vi "grabber_framescan.vi"() -> ()   [LabVIEW 2010]
uses:
  command_enum.ctl
  status_enum.ctl
  FPGAWrapperMH120124FrameScan_PXI7813R/settings_cluster_framescan.ctl
  common_typedefs/channels_cluster.ctl
  fpgaVIsAndControls/DDS_board_init_cluster.ctl
  fpgaVIsAndControls/gate_cluster.ctl
  common_typedefs/gate_parameters_cluster.ctl
  <vilib>/rvi/interface/nirviReadWriteControl/nirviReadWriteControl.xnode
  <vilib>/rvi/interface/common/niFpgaNodeNameForErrorReporting.ctl
  <vilib>/rvi/errors/niLvFpgaWhatHappensToTopLevelVI.ctl
  <vilib>/dex/Flush And Wait Empty Condition.ctl
  <vilib>/rvi/interface/nirviMethod/nirviMethod.xnode
  <vilib>/rvi/interface/nirviCloseFPGA/nirviCloseFPGA.xnode
  <vilib>/Utility/error.llb/Error Cluster From Error Code.vi
  <vilib>/rvi/errors/niLvFpgaAdjustHostInterfaceError.vi
  <vilib>/FPGAPlugInAG/Dynamic/niLvFpga_Close_Dynamic.vi
  NiFpgaLv.dll
panel:
  out "stop":bool
  out "read size":u32
  out "Elements Remaining 1":u32
  out "element":T1 {"DDS board initialization parameters"."Modus" scale=0.0..4.0}
  out "current status":T6
  out "pixel no.":i64
  out "last command_not_acq":T7
  out "FIFO overflow?":bool
  out "last command?":T7
  out "error out":errorcluster
  # "FSK"
  # "Ramped"
  # "FSK"
  # "Chirp Modus"
  # "Unramped"
  # "BPSK"
  # "Single Tone"
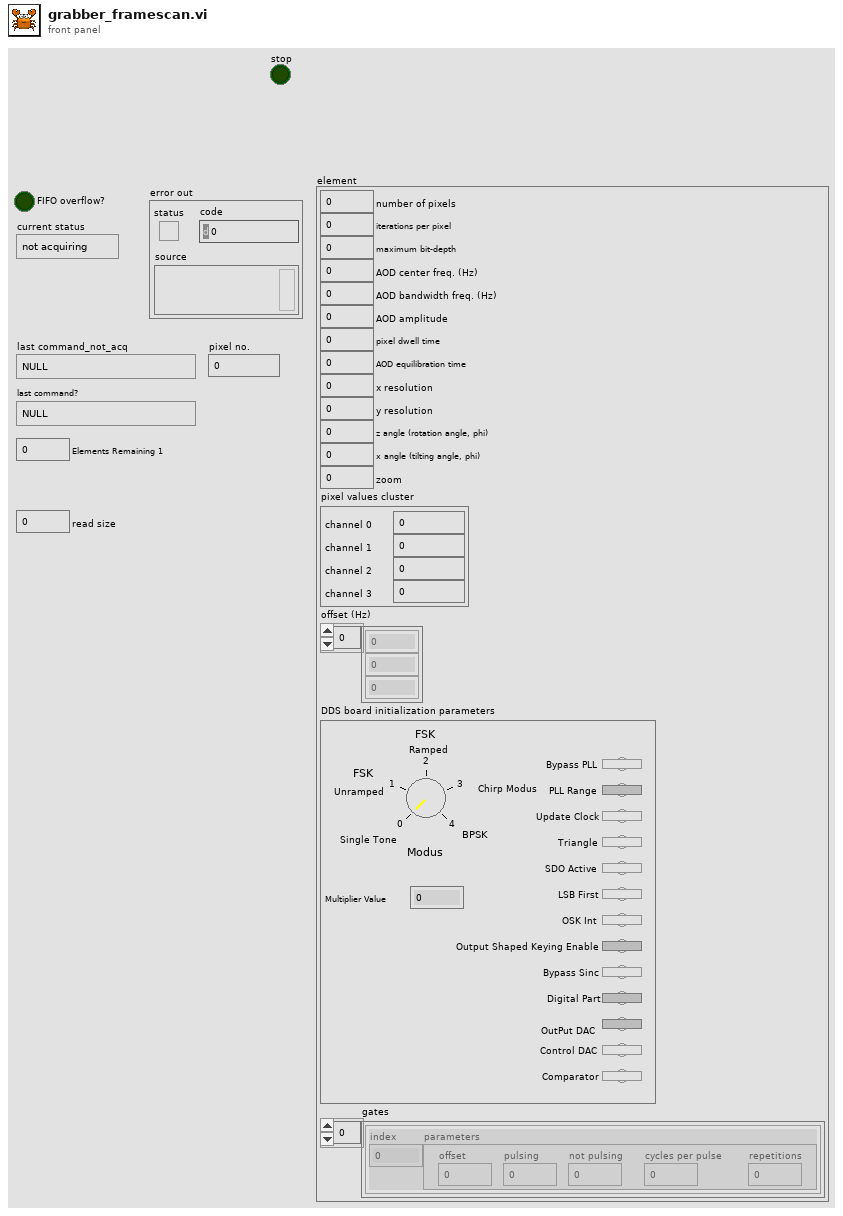
[diagram p1: front panel]
types:
  T1 = typedef "settings_cluster_framescan.ctl" = cluster{"number of pixels":i32, "iterations per pixel":i32, "maximum bit-depth":i8, "AOD center freq. (Hz)":dbl, "AOD bandwidth freq. (Hz)":dbl, "AOD amplitude":dbl, "pixel dwell time":dbl, "AOD equilibration time":dbl, "x resolution":i32, "y resolution":i32, "z angle (rotation angle, phi)":dbl, "x angle (tilting angle, phi)":dbl, "zoom":dbl, "pixel values cluster":T2, "offset (Hz)":dbl[], "DDS board initialization parameters":T3, "gates":T4[]}
  T2 = typedef "channels_cluster.ctl" = cluster{"channel 0":u32, "channel 1":u32, "channel 2":u32, "channel 3":u32}
  T3 = typedef "DDS_board_init_cluster.ctl" = cluster{"Bypass PLL":bool, "PLL Range":bool, "Update Clock":bool, "Triangle ":bool, "SDO Active":bool, "LSB First":bool, "OSK Int":bool, "Output Shaped Keying Enable":bool, "Bypass Sinc":bool, "Digital Part":bool, "OutPut DAC":bool, "Control DAC":bool, "Comparator":bool, "Modus":u8, "Multiplier Value":u8}
  T4 = typedef "gate_cluster.ctl" = cluster{"index":i32, "parameters":T5}
  T5 = typedef "gate_parameters_cluster.ctl" = cluster{"offset":i64, "pulsing":i64, "not pulsing":i64, "cycles per pulse":i64, "repetitions":i64}
  T6 = typedef "status_enum.ctl" = enum16{"not acquiring", "acquiring"}
  T7 = typedef "command_enum.ctl" = enum8{"NULL", "update", "start", "stop", "reset", "shut-down"}
  T8 = typedef "network_streaming_queues_cluster.ctl" = cluster{"command reader":refnum<k21>, "data writer":refnum<k21>, "raps reader":refnum<k21>, "settings framescan reader":refnum<k21>, "configuration framescan reader":refnum<k21>, "settings raps reader":refnum<k21>, "configuration raps reader":refnum<k21>, "update queue":refnum<queue>}
  T9 = typedef "niFpgaNodeNameForErrorReporting.ctl" = enum16{"Open FPGA VI Reference", "Read/Write Control", "Invoke Method: Abort", "Invoke Method: Acknowledge IRQ", "Invoke Method: Download", "Invoke Method: FIFO.Configure", "Invoke Method: FIFO.Read", "Invoke Method: FIFO.Start", "Invoke Method: FIFO.Stop", "Invoke Method: FIFO.Write", "Invoke Method: Reset", "Invoke Method: Run", "Invoke Method: Wait on IRQ", "Close FPGA VI Reference"}
  T10 = typedef "niLvFpgaWhatHappensToTopLevelVI.ctl" = enum16{"top level VI scripted behind XNode", "top level VI inlined behind XNode"}
  T11 = typedef "Flush And Wait Empty Condition.ctl" = u8
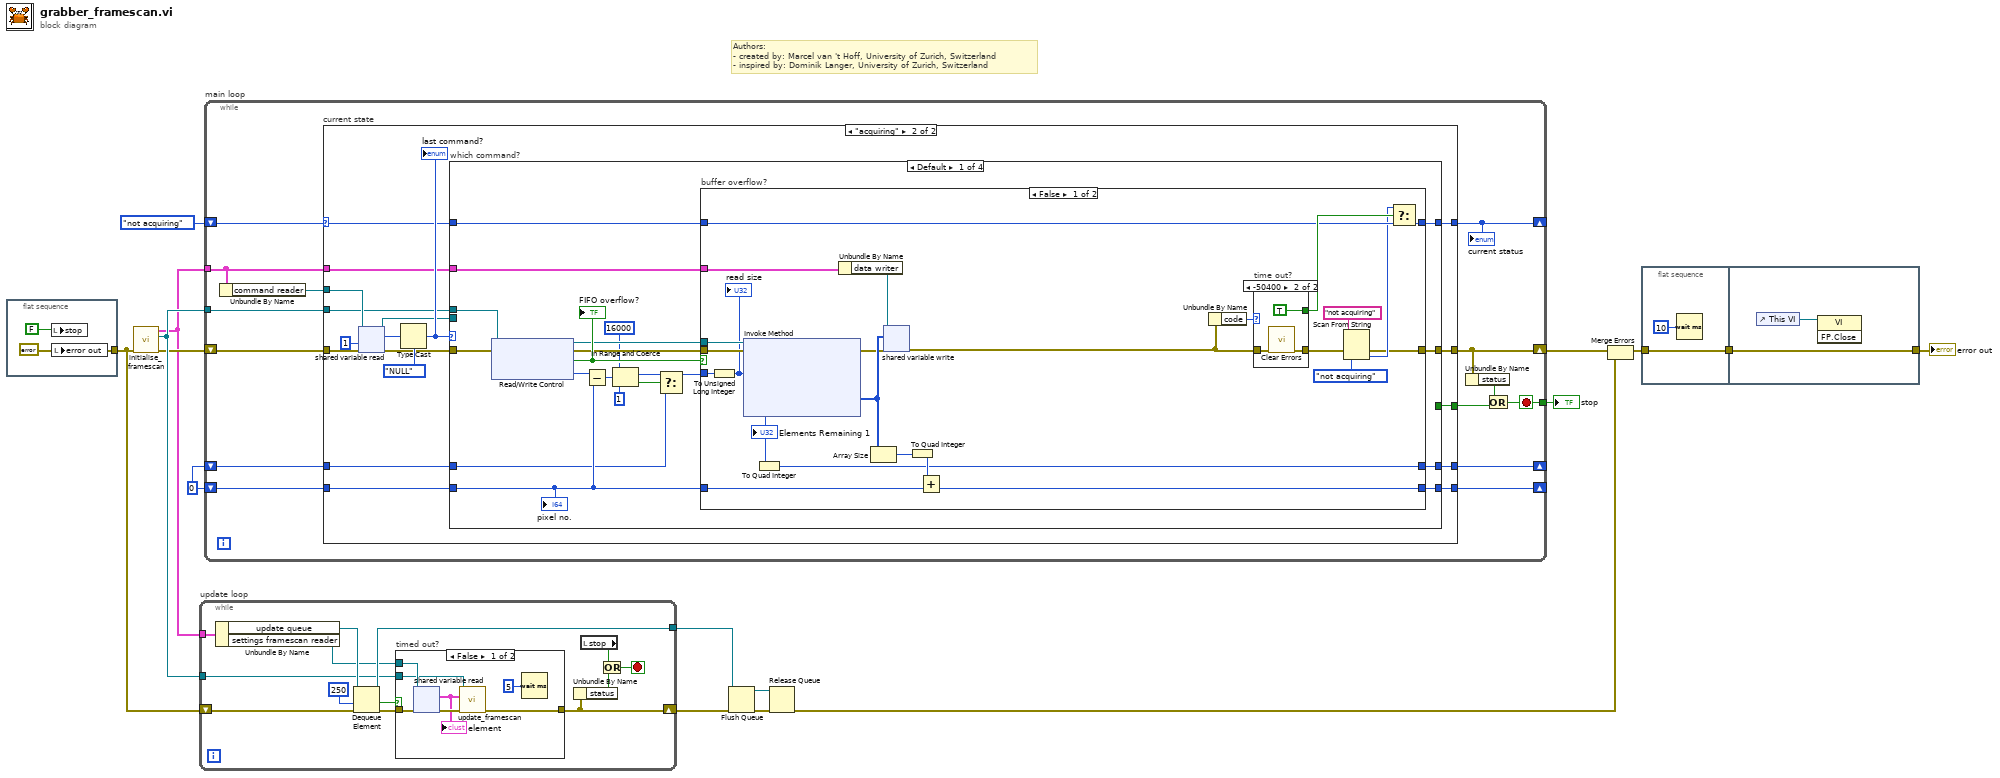
[diagram p0: block diagram]
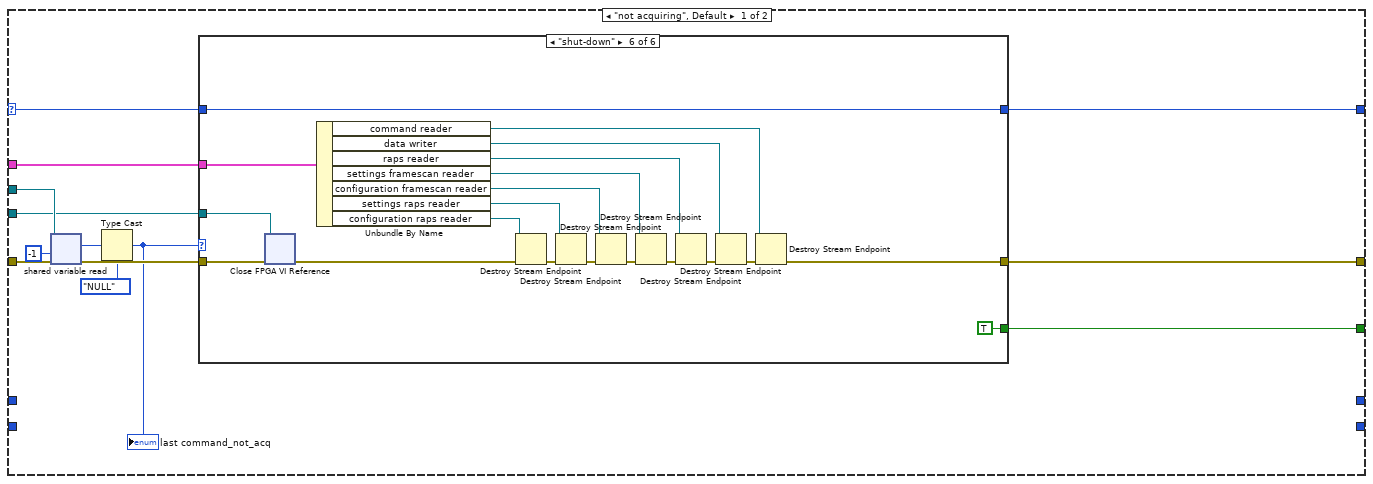
[diagram p3: hidden frame]
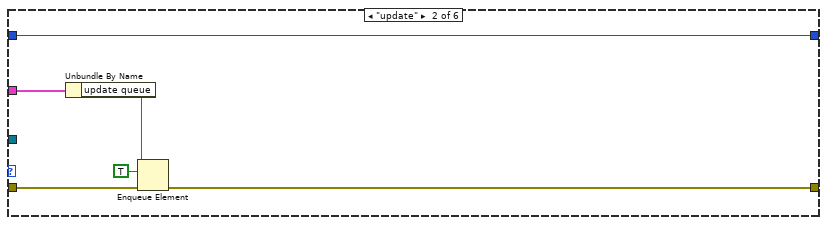
[diagram p5: hidden frame]
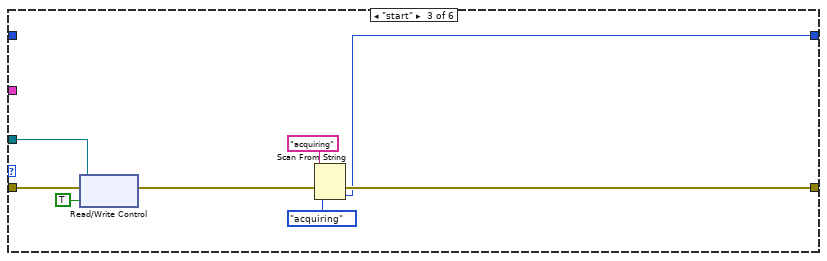
[diagram p6: hidden frame]
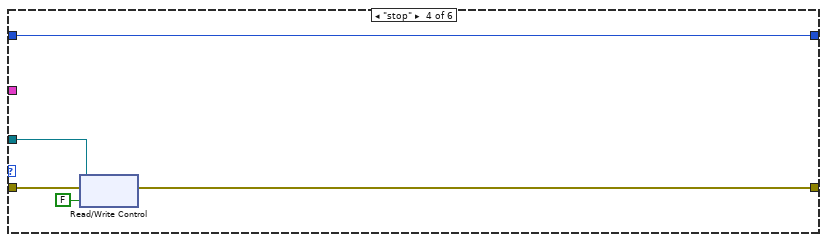
[diagram p7: hidden frame]
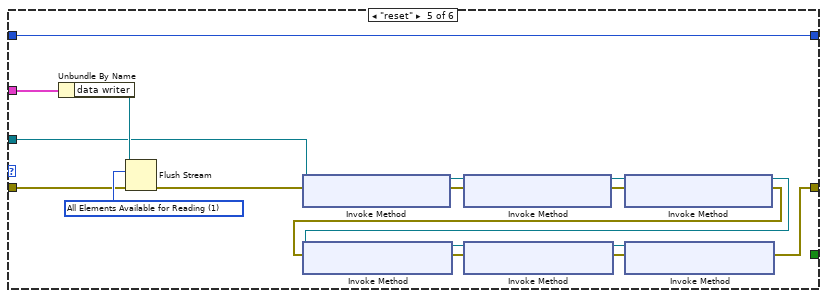
[diagram p8: hidden frame]
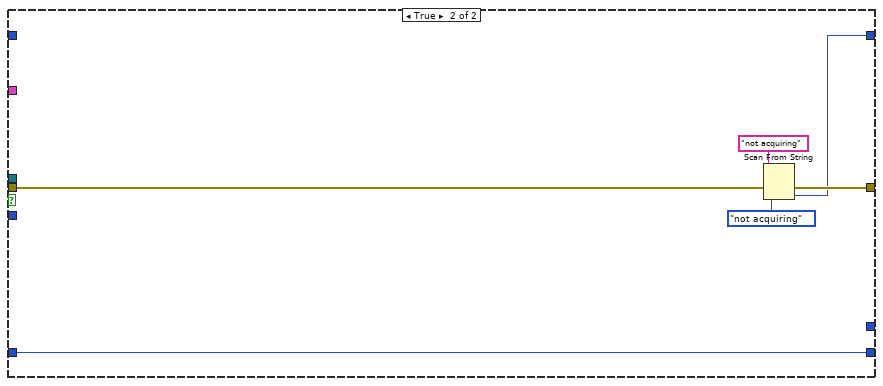
[diagram p10: hidden frame]
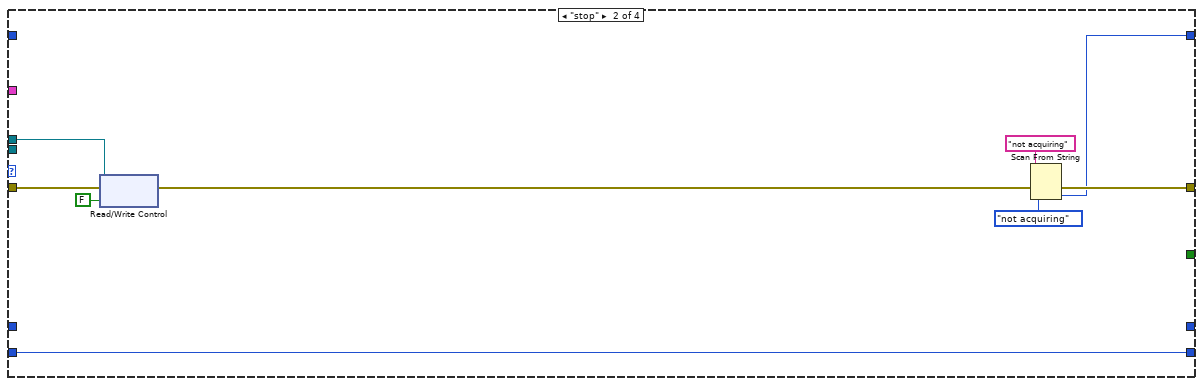
[diagram p11: hidden frame]
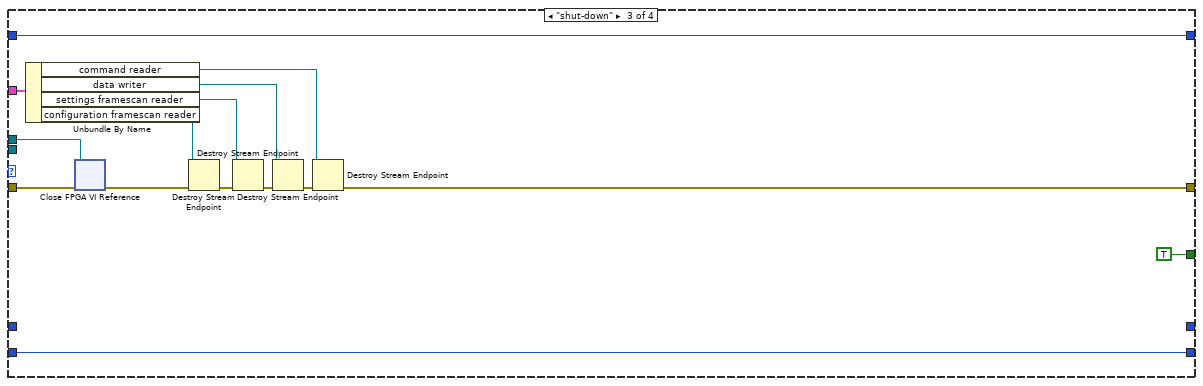
[diagram p12: hidden frame]
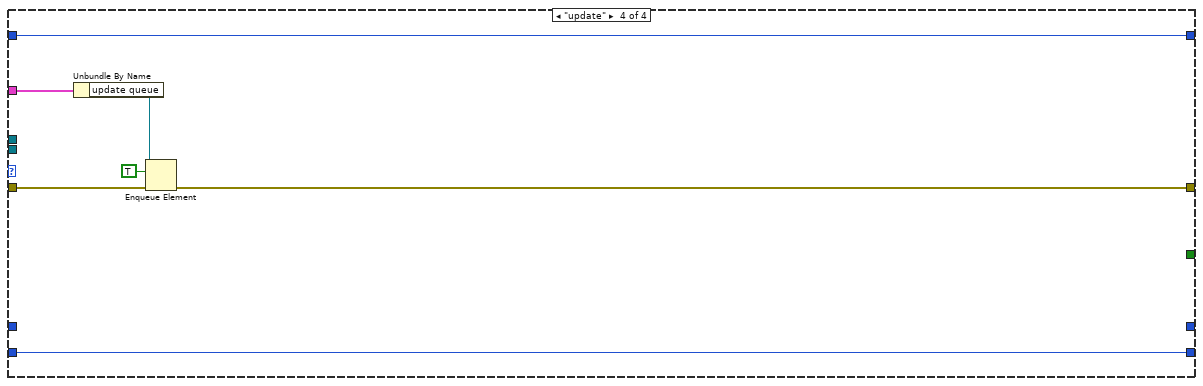
[diagram p13: hidden frame]
diagram:
  w1 = i64 0
  # "Authors:\n- created by: Marcel van 't Hoff, University of Zurich, Switzerland\n- inspired by: Dominik Langer, University of Zurich, Switzerland"
  n1 = flat-sequence {
    tunnel: [w18] -> w2
    frame #0 {
      w18 = errorcluster {"status"=FALSE, "code"=0, "source"=""} ("error in (no error)")
      n2 = local write "stop"(FALSE ("stop")) -> ()
      n3 = local write "error out"(w18) -> ()
    }
  }
  n4 = call "initialise_framescan.vi"("error in (no error)"=w2) -> ("error out"=w13:errorcluster, "FPGA VI Reference Out"=w14:refnum<k20>, "network streaming queues out"=w3:T8)  [unwired: 8 in]
  n5 = while "update loop" {
    tunnel: w14 -> [w19]
    tunnel: w3 -> [w31]
    tunnel: [w24] -> w11
    shift-right: [w30] -> w8
    shift-left: w2 -> [w26]
    stop <- w27 stop-if-true
    n6 = Unbundle By Name(w31) -> ("update queue"=w25:refnum<queue>, "settings framescan reader"=w23:refnum<k21>)
    n7 = Dequeue Element(queue=w25, timeout in ms (-1)=250, error in (no error)=w26) -> (queue out=w24:refnum<queue>, timed out?=w20:bool, error out=w21:errorcluster)  [unwired: 1 out]
    n8 = case "timed out?" shown="False" w20 {
      tunnel: w23 -> [w38 _]
      tunnel: w19 -> [w36 _]
      tunnel: [w35 w39] -> w30
      tunnel: w21 -> [w33 w39]
      frame False {
        n9 = shared-variable-read(w38, w33) -> (w37:errorcluster, w32:T1)  [unwired: 1 in, 2 out]
        "element" <- w32
        n10 = call "update_framescan.vi"("error in (no error)"=w37, "settings cluster"=w32, "FPGA VI Reference In"=w36) -> ("error out"=w35:errorcluster)  [unwired: 8 in]
        n11 = Wait (ms)(milliseconds to wait=u32 5) -> ()  [unwired: 1 out]
      }
      frame True {
      }
    }
    n12 = Unbundle By Name(w30) -> ("status"=w29:bool)
    n13 = local read "stop"() -> (w28:bool)
    n14 = Or(x=w28, y=w29) -> (x .or. y?=w27:bool)
  }
  n15 = while "main loop" {
    tunnel: w14 -> [w50]
    tunnel: w3 -> [w51]
    shift-right: [w46] -> _
    shift-left: status_enum."not acquiring" ("status enum") -> [w53]
    shift-right: [w45] -> w6
    shift-left: w13 -> [w49]
    shift-right: [w47] -> _
    shift-left: w1 -> [w48]
    tunnel: [w42] -> w12
    shift-right: [w41] -> _
    shift-left: w1 -> [w40]
    stop <- w42 stop-if-true
    n16 = Unbundle By Name(w51) -> ("command reader"=w52:refnum<k21>)
    n17 = case "current state" shown="\"acquiring\"" w53 {
      selector: w53 -> [w60 w239]
      tunnel: w52 -> [w65 w245]
      tunnel: w51 -> [w62 w240]
      tunnel: w50 -> [w63 w238]
      tunnel: w49 -> [w66 w244]
      tunnel: w48 -> [_ w237]
      tunnel: [_ w236] -> w47
      tunnel: [w59 w235] -> w45
      tunnel: [w61 w234] -> w46
      tunnel: [w58 w230] -> w43
      tunnel: [_ w229] -> w41
      tunnel: w40 -> [_ w228]
      frame "not acquiring", Default {
        n18 = shared-variable-read(w65, w66, -1 ("timeout in ms (-1)")) -> (w64:errorcluster, w55:u8)  [unwired: 2 out]
        n19 = Type Cast(type=command_enum."NULL" ("command"), x=w55) -> (*(type *) &x=w56:T7)
        "last command_not_acq" <- w56
        n20 = case shown="\"shut-down\"" w56 {
          tunnel: w64 -> [w67 w71 w82 w125 w166 w221]
          tunnel: w63 -> [_ _ w80 w126 w167 w220]
          tunnel: w62 -> [_ w70 _ _ w183 w217]
          tunnel: [w68 w74 w75 w122 w168 w218] -> w61
          tunnel: w60 -> [w68 w74 _ w122 w168 w218]
          tunnel: [w67 w69 w78 w123 w169 w203] -> w59
          tunnel: [_ _ _ _ _ TRUE] -> w58
          frame "NULL", Default {
          }
          frame "update" {
            n21 = Unbundle By Name(w70) -> ("update queue"=w73:refnum<queue>)
            n22 = Enqueue Element(queue=w73, element=TRUE, error in (no error)=w71) -> (error out=w69:errorcluster)  [unwired: 1 in, 2 out]
          }
          frame "start" {
            n23 = xnode "Read/Write Control"("FPGA VI Reference In"=w80, "error in"=w82, "acquire?"=TRUE) -> ("error out"=w79:errorcluster)  [unwired: 1 out]
            n24 = Scan From String(input string="acquiring", error in=w79, default 1=status_enum."acquiring" ("status enum")) -> (error out=w78:errorcluster, output 1=w75:T6)  [unwired: 2 in, 2 out]
          }
          frame "stop" {
            n25 = xnode "Read/Write Control"("FPGA VI Reference In"=w126, "error in"=w125, "acquire?"=FALSE) -> ("error out"=w123:errorcluster)  [unwired: 1 out]
          }
          frame "reset" {
            w181 = T11 1 items=["All Elements Read From Stream", "All Elements Available for Reading"] ("wait condition")
            n26 = Unbundle By Name(w183) -> ("data writer"=w182:refnum<k21>)
            n27 = Flush Stream(8:w166, 10:w181, 11:w182) -> (0:w180:errorcluster)  [unwired: 1 in, 2 out]
            n28 = xnode "Invoke Method"("FPGA VI Reference In"=w167, "error in"=w180) -> ("FPGA VI Reference Out"=w176:refnum<k20>, "error out"=w179:errorcluster)
            n29 = xnode "Invoke Method"("FPGA VI Reference In"=w176, "error in"=w179) -> ("FPGA VI Reference Out"=w177:refnum<k20>, "error out"=w178:errorcluster)
            n30 = xnode "Invoke Method"("FPGA VI Reference In"=w177, "error in"=w178) -> ("FPGA VI Reference Out"=w175:refnum<k20>, "error out"=w172:errorcluster)
            n31 = xnode "Invoke Method"("FPGA VI Reference In"=w175, "error in"=w172) -> ("FPGA VI Reference Out"=w173:refnum<k20>, "error out"=w174:errorcluster)
            n32 = xnode "Invoke Method"("FPGA VI Reference In"=w173, "error in"=w174) -> ("FPGA VI Reference Out"=w170:refnum<k20>, "error out"=w171:errorcluster)
            n33 = xnode "Invoke Method"("FPGA VI Reference In"=w170, "error in"=w171) -> ("error out"=w169:errorcluster)  [unwired: 1 out]
          }
          frame "shut-down" {
            n34 = xnode "Close FPGA VI Reference"("FPGA VI Reference In"=w220, "error in"=w221) -> ("error out"=w202:errorcluster)
            n35 = Unbundle By Name(w217) -> ("command reader"=w216:refnum<k21>, "data writer"=w210:refnum<k21>, "raps reader"=w211:refnum<k21>, "settings framescan reader"=w212:refnum<k21>, "configuration framescan reader"=w213:refnum<k21>, "settings raps reader"=w214:refnum<k21>, "configuration raps reader"=w215:refnum<k21>)
            n36 = Destroy Stream Endpoint(8:w202, 11:w215) -> (0:w209:errorcluster)
            n37 = Destroy Stream Endpoint(8:w209, 11:w214) -> (0:w208:errorcluster)
            n38 = Destroy Stream Endpoint(8:w208, 11:w213) -> (0:w207:errorcluster)
            n39 = Destroy Stream Endpoint(8:w207, 11:w212) -> (0:w206:errorcluster)
            n40 = Destroy Stream Endpoint(8:w206, 11:w211) -> (0:w205:errorcluster)
            n41 = Destroy Stream Endpoint(8:w205, 11:w210) -> (0:w204:errorcluster)
            n42 = Destroy Stream Endpoint(8:w204, 11:w216) -> (0:w203:errorcluster)
          }
        }
      }
      frame "acquiring" {
        n43 = shared-variable-read(w245, w244, 1 ("timeout in ms (-1)")) -> (w232:refnum<k21>, w241:errorcluster, w233:u8)  [unwired: 1 out]
        n44 = Type Cast(type=command_enum."NULL" ("command"), x=w233) -> (*(type *) &x=w242:T7)
        "last command?" <- w242
        n45 = case "which command?" shown="Default" w242 {
          tunnel: w241 -> [w264 w454 w511 w519]
          tunnel: w240 -> [w259 _ w501 w522]
          tunnel: w239 -> [w255 _ w509 w523]
          tunnel: w238 -> [w265 w457 w510 _]
          tunnel: w237 -> [w257 w455 w504 w524]
          tunnel: [w258 w455 w504 w524] -> w236
          tunnel: [w256 w450 w508 w518] -> w235
          tunnel: [w254 w449 w509 w523] -> w234
          tunnel: w232 -> [_ _ _ _]
          tunnel: [_ _ TRUE _] -> w230
          tunnel: [w250 _ _ _] -> w229
          tunnel: w228 -> [w248 _ _ _]
          frame Default {
            n46 = xnode "Read/Write Control"("FPGA VI Reference In"=w265, "error in"=w264) -> ("FPGA VI Reference Out"=w261:refnum<k20>, "error out"=w260:errorcluster, "FIFO_DMA full?"=w263:bool, "current pixel no."=w262:i64)
            "FIFO overflow?" <- w263
            n47 = Subtract(x=w262, y=w257) -> (x-y=w252:i64)
            n48 = In Range and Coerce(upper limit=i64 16000, x=w252, lower limit=i64 1) -> (coerced(x)=w247:i64, In Range?=w249:bool)
            n49 = Select(t=w247, s=w249, f=w248) -> (s? t:f=w246:i64)
            n50 = case "buffer overflow?" shown="False" w263 {
              tunnel: w246 -> [w288 _]
              tunnel: w261 -> [w289 _]
              tunnel: w260 -> [w285 w369]
              tunnel: w259 -> [w287 _]
              tunnel: [w282 w372] -> w258
              tunnel: w257 -> [w281 w372]
              tunnel: [w268 w368] -> w256
              tunnel: w255 -> [w278 _]
              tunnel: [w277 w367] -> w254
              tunnel: [w274 _] -> w250
              frame False {
                n51 = To Unsigned Long Integer(number=w288) -> (unsigned 32bit integer=w276:u32)
                "read size" <- w276
                n52 = xnode "Invoke Method"("FPGA VI Reference In"=w289, "error in"=w285, "Number of Elements"=w276) -> ("error out"=w267:errorcluster, "Data"=w273:u64[], "Elements Remaining"=w275:u32)  [unwired: 1 in, 1 out]
                "Elements Remaining 1" <- w275
                n53 = To Quad Integer(1:w275) -> (0:w274:i64)
                n54 = Unbundle By Name(w287) -> ("data writer"=w286:refnum<k21>)
                n55 = Array Size(array=w273) -> (size(s)=w284:i32)
                n56 = shared-variable-write(w286, w267, w273) -> (w266:errorcluster)  [unwired: 1 in, 2 out]
                n57 = To Quad Integer(1:w284) -> (0:w283:i64)
                n58 = Add(x=w283, y=w281) -> (x+y=w282:i64)
                n59 = Unbundle By Name(w266) -> ("code"=w280:i32)
                n60 = case "time out?" shown="-50400" w280 {
                  tunnel: w266 -> [w290 w293]
                  tunnel: [w290 w292] -> w269
                  tunnel: [_ TRUE] -> w279
                  frame Default {
                  }
                  frame -50400 {
                    n61 = call <vilib>:"Clear Errors.vi"("error in (no error)"=w293) -> ("error out"=w292:errorcluster)  [unwired: 6 in]
                  }
                }
                n62 = Scan From String(input string="not acquiring", error in=w269, default 1=status_enum."not acquiring" ("status enum")) -> (error out=w268:errorcluster, output 1=w270:T6)  [unwired: 2 in, 2 out]
                n63 = Select(t=w270, s=w279, f=w278) -> (s? t:f=w277:T6)
              }
              frame True {
                n64 = Scan From String(input string="not acquiring", error in=w369, default 1=status_enum."not acquiring" ("status enum")) -> (error out=w368:errorcluster, output 1=w367:T6)  [unwired: 2 in, 2 out]
              }
            }
            "pixel no." <- w257
          }
          frame "stop" {
            n65 = xnode "Read/Write Control"("FPGA VI Reference In"=w457, "error in"=w454, "acquire?"=FALSE) -> ("error out"=w451:errorcluster)  [unwired: 1 out]
            n66 = Scan From String(input string="not acquiring", error in=w451, default 1=status_enum."not acquiring" ("status enum")) -> (error out=w450:errorcluster, output 1=w449:T6)  [unwired: 2 in, 2 out]
          }
          frame "shut-down" {
            n67 = Unbundle By Name(w501) -> ("command reader"=w503:refnum<k21>, "data writer"=w502:refnum<k21>, "settings framescan reader"=w498:refnum<k21>, "configuration framescan reader"=w499:refnum<k21>)
            n68 = xnode "Close FPGA VI Reference"("FPGA VI Reference In"=w510, "error in"=w511) -> ("error out"=w500:errorcluster)
            n69 = Destroy Stream Endpoint(8:w500, 11:w499) -> (0:w507:errorcluster)
            n70 = Destroy Stream Endpoint(8:w507, 11:w498) -> (0:w497:errorcluster)
            n71 = Destroy Stream Endpoint(8:w497, 11:w502) -> (0:w506:errorcluster)
            n72 = Destroy Stream Endpoint(8:w506, 11:w503) -> (0:w508:errorcluster)
          }
          frame "update" {
            n73 = Unbundle By Name(w522) -> ("update queue"=w521:refnum<queue>)
            n74 = Enqueue Element(queue=w521, element=TRUE, error in (no error)=w519) -> (error out=w518:errorcluster)  [unwired: 1 in, 2 out]
          }
        }
      }
    }
    "current status" <- w46
    n75 = Unbundle By Name(w45) -> ("status"=w44:bool)
    n76 = Or(x=w44, y=w43) -> (x .or. y?=w42:bool)
  }
  "stop" <- w12
  n77 = Flush Queue(queue=w11, error in (no error)=w8) -> (queue out=w10:refnum<queue>, error out=w9:errorcluster)  [unwired: 1 out]
  n78 = Release Queue(queue=w10, error in (no error)=w9) -> (error out=w7:errorcluster)  [unwired: 1 in, 2 out]
  n79 = Merge Errors(w6, w7) -> (w5:errorcluster)
  n80 = flat-sequence {
    tunnel: w5 -> [w526]
    tunnel: [w526] -> w4
    tunnel: [w528] -> w15
    tunnel: w4 -> [w528]
    frame #0 {
      n81 = Wait (ms)(milliseconds to wait=u32 10) -> ()  [unwired: 1 out]
    }
    frame #1 {
      n82 = control-ref of="This VI"() -> (w527:refnum<vi>)
      n83 = invoke class="VI" method="FP.Close"(reference=w527) -> ()  [unwired: 2 in, 3 out]
    }
  }
  "error out" <- w15
